vi "Frame Wall Set.vi"(8 "error in (no error)":errorcluster, 9 "Wall Stiffness":dbl=0.2 format="%#.1f", 10 "Restrict to Frame":bool=TRUE) -> (0 "error out":errorcluster)   [LabVIEW 2019, in "Haptic Prog Interface.lvlib"]
doc: "Returns the horizontal xy-position of the haptic pen in nm, and the vertical z-position in mm. The horizontal position depends on the frame origin and frame size.\n\n<b>Position:</b> Returns a cluster of the x (nm), y (nm), and z (mm) positions of the pen."
uses:
  Haptic Prog Interface.lvlib
  dll_path.vi
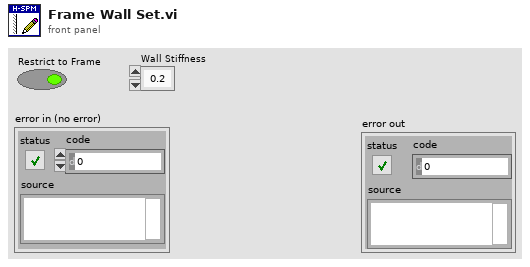
[diagram p1: front panel]
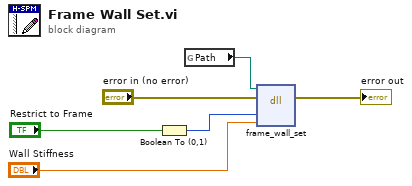
[diagram p0: block diagram]
diagram:
  n1 = Boolean To (0,1)(Boolean="Restrict to Frame") -> (0, 1=w3:i16)
  n2 = global read "dll_path.vi" "Path"() -> (w6:path)
  n3 = dll-call lib="C:/Users/freem/Documents/GitHub/HapticSPM/Haptic-Programming-Interface/x64/Release/Haptic Programming Interface.dll" fn="frame_wall_set"(path in=w6, error in="error in (no error)", "input"=w3, "k_wall"="Wall Stiffness") -> (error out=→"error out":errorcluster)  [unwired: 4 in, 1 out]
